vi "MTS_PreapareImage.vi"(0 "WS File Tree":refnum<vi>, 1 "Info":string, 5 "Workspace":path, 7 "Measurement Type":T3(ring), 9 "Image Measurent Parameters":T1, 11 "error in":errorcluster, 12 "Trigger":dbl[](array[numeric])) -> (4 "File Name (dup)":path, 6 "File No":i32, 8 "Image Header":T2, 10 "Comment":string, 15 "error out":errorcluster)   [LabVIEW 2011]
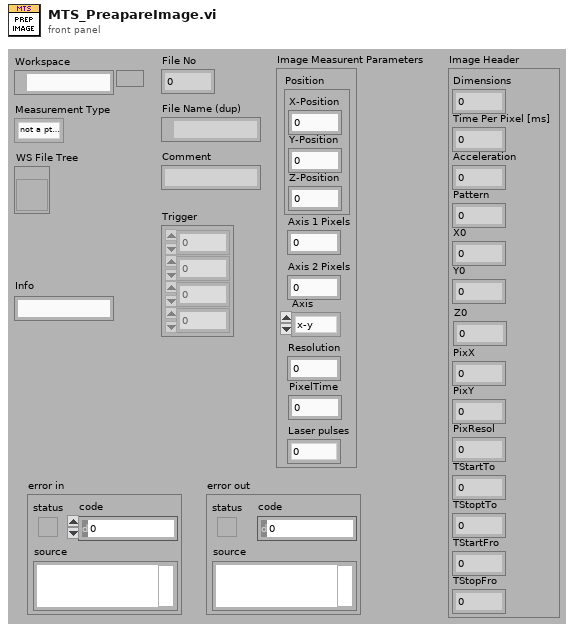
[diagram p1: front panel]
types:
  T1 = cluster{"Position":cluster{"X-Position":dbl, "Y-Position":dbl, "Z-Position":dbl}, "Axis 1 Pixels":u16, "Axis 2 Pixels":u16, "Axis":enum16{"x-y", "x-z", "y-x", "y-z", "z-x", "z-y"}, "Resolution":dbl, "PixelTime":dbl, "Laser pulses":i32}
  T2 = cluster{"Dimensions":i32, "Time Per Pixel [ms]":dbl, "Acceleration":i32, "Pattern":i32, "X0":sgl, "Y0":sgl, "Z0":dbl, "PixX":i32, "PixY":i32, "PixResol":sgl, "TStartTo":sgl, "TStoptTo":sgl, "TStartFro":sgl, "TStopFro":sgl}
  T3 = enum16{"not a pt3 File", "Image File", "Point Measurement", "Auto Point", "Line Scan"}
  T4 = enum16{"unknown", "pt3 File", "png Image", "bmp Image"}
  T5 = cluster{"X-Position":dbl, "Y-Position":dbl, "Z-Position":dbl}
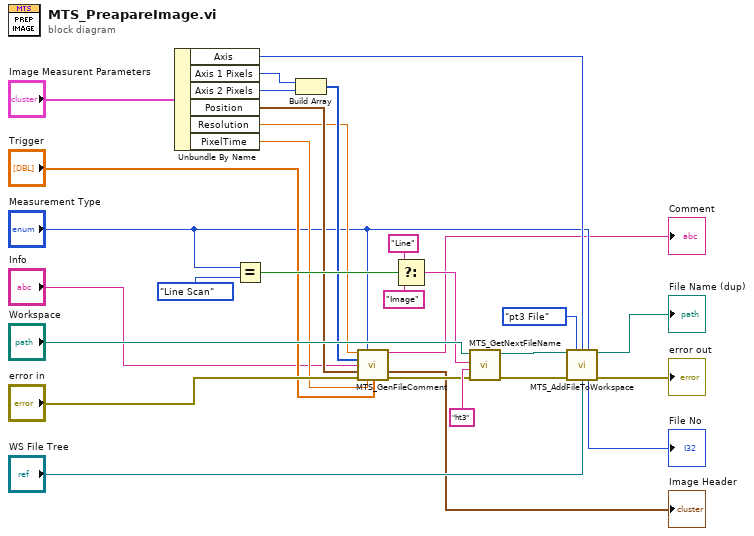
[diagram p0: block diagram]
diagram:
  n1 = Unbundle By Name("Image Measurent Parameters") -> ("Axis"=w17:enum16{"x-y", "x-z", "y-x", "y-z", "z-x", "z-y"}, "Axis 1 Pixels"=w18:u16, "Axis 2 Pixels"=w19:u16, "Position"=w8:T5, "Resolution"=w4:dbl, "PixelTime"=w5:dbl)
  n2 = Equal?(x="Measurement Type", y=T3."Line Scan" ("Measurement Type")) -> (x = y?=w15:bool)
  n3 = Build Array(w18, w19) -> (w7:u16[])
  n4 = call "MTS_GenFileComment.vi"("Resolution"=w4, "Measurement Type"="Measurement Type", "Pixels"=w7, "Info"="Info", "Upper Left"=w8, "error in"="error in", "Time Per Pixel [ms]"=w5, "Trigger"="Trigger") -> ("Comment"=→"Comment":string, "Image Header"=→"Image Header":T2, "error out"=w10:errorcluster)  [unwired: 4 in, 1 out]
  n5 = Select(t="Line" ("Measurement Type"), s=w15, f="Image" ("Measurement Type")) -> (s? t:f=w14:string)
  n6 = call "MTS_GetNextFileName.vi"("error in (no error)"=w10, "File Type"="ht3", "Measurement Type"=w14, "Workspace"="Workspace") -> ("error out"=w23:errorcluster, "Next File Name"=w24:path)  [unwired: 6 in]
  n7 = call "MTS_AddFileToWorkspace.vi"("File Name"=w24, "File Type"=T4."pt3 File", "Scan Axis"=w17, "Measurement Type"="Measurement Type", "error in (no error)"=w23, "Tree Refnum"="WS File Tree") -> ("File Name (dup)"=→"File Name (dup)":path, "File No"=→"File No":i32, "error out"=→"error out":errorcluster)  [unwired: 7 in]
